vi "P4CMD Dialog - Adv Config Options.vi"(8 "error in (no error)":errorcluster, 9 "adv cfg options in":T1) -> (0 "error out":errorcluster, 1 "adv cfg  options out":T1, 3 "cancelled?":bool)   [LabVIEW 2017, in "NI_SCC_P4CMD.lvlib"]
uses:
  <vilib>/SourceControl/Providers/P4CMD/NI_SCC_P4CMD.lvlib
  <vilib>/SourceControl/Providers/P4CMD/P4CMD Advanced Options.ctl
panel:
  in  "supress dlgs?":bool
  in  "Lock?":bool=TRUE
  in  "OK":bool
  in  "Cancel":bool
  in  "Help":bool
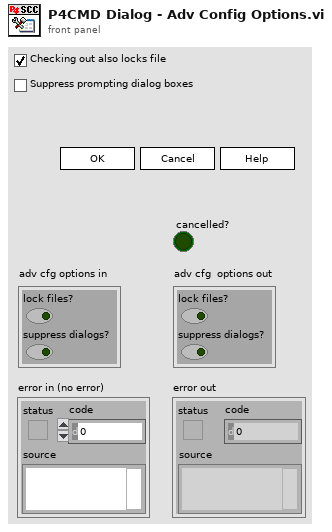
[diagram p1: front panel]
types:
  T1 = typedef "NI_SCC_P4CMD.lvlib/P4CMD Advanced Options.ctl" = cluster{"lock files?":bool, "suppress dialogs?":bool}
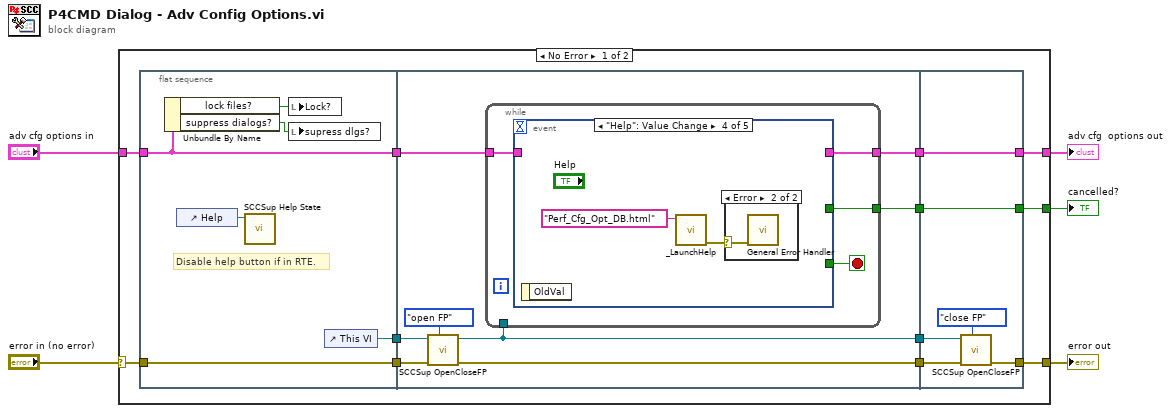
[diagram p0: block diagram]
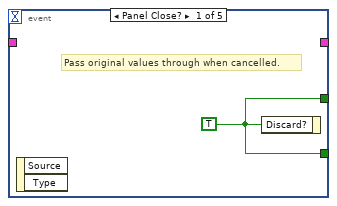
[diagram p2: hidden frame]
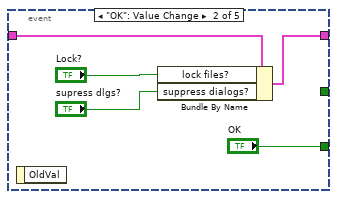
[diagram p3: hidden frame]
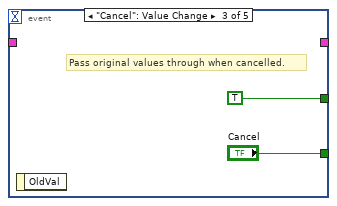
[diagram p4: hidden frame]
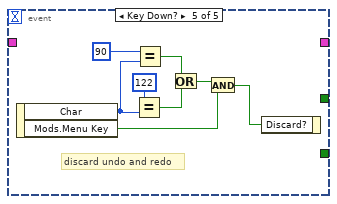
[diagram p6: hidden frame]
diagram:
  n1 = case shown="No Error" "error in (no error)" {
    selector: "error in (no error)" -> [w15 w62]
    tunnel: [w12 w62] -> w4
    tunnel: "adv cfg options in" -> [w10 w61]
    tunnel: [w7 w61] -> w2
    tunnel: [w6 _] -> w1
    frame No Error {
      n2 = flat-sequence {
        tunnel: [w19] -> w17
        tunnel: w15 -> [w20]
        tunnel: [w20] -> w14
        tunnel: [w21] -> w11
        tunnel: w10 -> [w21]
        tunnel: [w29] -> w16
        tunnel: w17 -> [w30]
        tunnel: w14 -> [w28]
        tunnel: [w27] -> w13
        tunnel: w11 -> [w26]
        tunnel: [w25] -> w9
        tunnel: [w24] -> w8
        tunnel: w16 -> [w59]
        tunnel: w13 -> [w58]
        tunnel: [w57] -> w12
        tunnel: [w56] -> w7
        tunnel: w9 -> [w56]
        tunnel: [w55] -> w6
        tunnel: w8 -> [w55]
        frame #0 {
          # "Disable help button if in RTE."
          n3 = Unbundle By Name(w21) -> ("lock files?"=w23:bool, "suppress dialogs?"=w22:bool)
          n4 = control-ref of="Help"() -> (w18:refnum<vi>)
          n5 = call <vilib>:"SCCSup Help State.vi"("help ref"=w18) -> ()  [unwired: 10 in, 1 out]
          n6 = local write "Lock?"(w23) -> ()
          n7 = local write "supress dlgs?"(w22) -> ()
          n8 = control-ref of="This VI"() -> (w19:refnum<vi>)
        }
        frame #1 {
          n9 = call <vilib>:"SCCSup OpenCloseFP.vi"("function"=enum16{"open FP", "close FP"}."open FP", "error in (no error)"=w28, "VI Refnum in"=w30) -> ("error out"=w27:errorcluster, "VI Refnum out"=w29:refnum<vi>)  [unwired: 7 in]
          n10 = while {
            tunnel: [w34] -> w24
            tunnel: w29 -> [_]
            tunnel: w26 -> [w33]
            tunnel: [w32] -> w25
            stop <- w35 stop-if-true
            n11 = event shown="[3] \"Help\": Value Change" {
              selector: _ -> [_ _ _ _ _]
              dyn-events: _ -> [_ _ _ _ _]
              timeout: _ -> [_ _ _ _ _]
              tunnel: [w36 "OK" "Cancel" _ _] -> w35
              tunnel: [w36 _ TRUE _ _] -> w34
              tunnel: w33 -> [_ w40 _ _ _]
              tunnel: [_ w37 _ _ _] -> w32
              event Panel Close? {
                w36 = TRUE
                # "Pass original values through when cancelled."
                n12 = event-data() -> ()  [unwired: 1 in, 2 out]
                n13 = event-data("Discard?"=w36) -> ()  [unwired: 1 in, 1 out]
              }
              event "OK": Value Change {
                n14 = event-data() -> ()  [unwired: 1 in, 1 out]
                n15 = Bundle By Name(cluster=w40, "lock files?"="Lock?", "suppress dialogs?"="supress dlgs?") -> (w37:T1)
              }
              event "Cancel": Value Change {
                # "Pass original values through when cancelled."
                n16 = event-data() -> ()  [unwired: 1 in, 1 out]
              }
              event "Help": Value Change {
                n17 = event-data() -> ()  [unwired: 1 in, 1 out]
                n18 = call <helpdir>:"_LaunchHelp.vi"("HTML filename"="Perf_Cfg_Opt_DB.html" ("Help topic")) -> ("error out"=w45:errorcluster)  [unwired: 6 in]
                n19 = case shown="Error" w45 {
                  selector: w45 -> [_ w46]
                  frame No Error {
                  }
                  frame Error {
                    n20 = call <vilib>:"General Error Handler.vi"("error in (no error)"=w46) -> ()  [unwired: 10 in, 5 out]
                  }
                }
              }
              event Key Down? {
                # "discard undo and redo"
                n21 = event-data() -> ("Char"=w49:i16, "Mods.Menu Key"=w48:bool)  [unwired: 1 in]
                n22 = Equal?(x=i16 122, y=w49) -> (x = y?=w52:bool)
                n23 = Equal?(x=i16 90, y=w49) -> (x = y?=w51:bool)
                n24 = Or(x=w51, y=w52) -> (x .or. y?=w50:bool)
                n25 = And(x=w50, y=w48) -> (x .and. y?=w47:bool)
                n26 = event-data("Discard?"=w47) -> ()  [unwired: 1 in, 1 out]
              }
            }
          }
        }
        frame #2 {
          n27 = call <vilib>:"SCCSup OpenCloseFP.vi"("function"=enum16{"open FP", "close FP"}."close FP", "error in (no error)"=w58, "VI Refnum in"=w59) -> ("error out"=w57:errorcluster)  [unwired: 7 in, 1 out]
        }
      }
    }
    frame Error {
    }
  }
  "error out" <- w4
  "cancelled?" <- w1
  "adv cfg  options out" <- w2
